vi "Zaber Beginner - Send a List of Commands.vi"() -> ()   [LabVIEW 2020]
doc: "The simplest VI you can write is just a list of commands with no logic. The block diagram makes a request, waits for the response, and then makes the next request until it gets to the end of the list.\nConnect your Zaber device to power and a serial port, then select the serial port on the front panel. Click the Run arrow, and the device will\ntake 5 steps backwards, and then extend back to where it started. The device has to start at least 50000 microsteps away from the home\nposition, so if you receive error response 21, just extend the device before running the VI. All commands are sent to Zaber device number 1."
uses:
  Public/Utility/Request.ctl
  ZaberTSeries.lvlib
panel:
  in  "VISA resource name":refnum<visa-resource-name>
  # "Connect your Zaber device to power and a serial port, then select the\nserial port below. Click the Run arrow above, and the device will\ntake 5 steps backwards, and then extend back to where it started. \nThe device has to start at least 500 microsteps away from the home\nposition, so if you receive error response 21, just extend the device\nbefore running the VI. All commands are sent to Zaber device number 1.\nType Ctrl-E to see how the block diagram is wired."
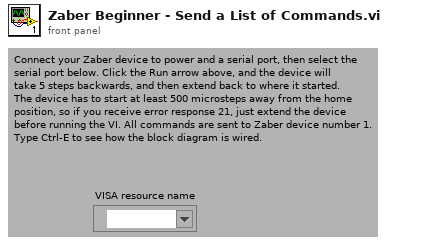
[diagram p1: front panel]
types:
  T1 = typedef "ZaberTSeries.lvlib/Request.ctl" = cluster{"Device Number":u8, "Command":u8, "Data":i32, "Response Count":i32}
  T2 = cluster{"Device Number":u8, "Command":u8, "Data":i32, "Response Count":i32}
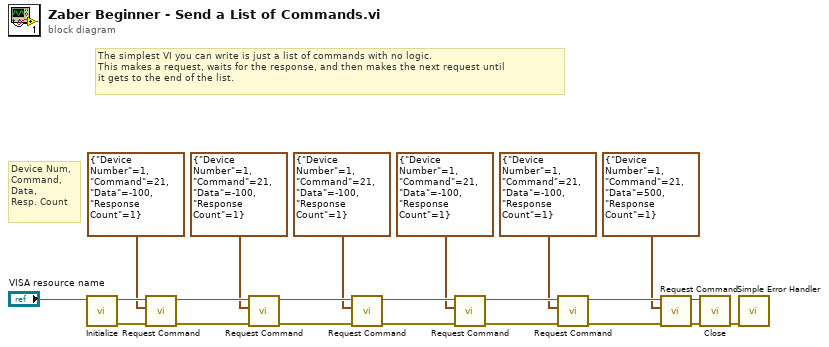
[diagram p0: block diagram]
diagram:
  # "The simplest VI you can write is just a list of commands with no logic.\nThis makes a request, waits for the response, and then makes the next request until\nit gets to the end of the list."
  # "Device Num,\nCommand,\nData,\nResp. Count"
  n1 = call "Initialize.vi"("VISA resource name"="VISA resource name") -> ("error out"=w22:errorcluster, "VISA resource name out"=w19:refnum<visa-resource-name>)  [unwired: 8 in, 1 out]
  n2 = call "Request Command.vi"("error in (no error)"=w22, "Request"=T2 {"Device Number"=1, "Command"=21, "Data"=-100, "Response Count"=1}, "VISA resource name"=w19) -> ("error out"=w21:errorcluster, "VISA resource name out"=w18:refnum<visa-resource-name>)  [unwired: 5 in, 2 out]
  n3 = call "Request Command.vi"("error in (no error)"=w21, "Request"=T1 {"Device Number"=1, "Command"=21, "Data"=-100, "Response Count"=1}, "VISA resource name"=w18) -> ("error out"=w7:errorcluster, "VISA resource name out"=w16:refnum<visa-resource-name>)  [unwired: 5 in, 2 out]
  n4 = call "Request Command.vi"("error in (no error)"=w7, "Request"=T1 {"Device Number"=1, "Command"=21, "Data"=-100, "Response Count"=1}, "VISA resource name"=w16) -> ("error out"=w8:errorcluster, "VISA resource name out"=w15:refnum<visa-resource-name>)  [unwired: 5 in, 2 out]
  n5 = call "Request Command.vi"("error in (no error)"=w8, "Request"=T1 {"Device Number"=1, "Command"=21, "Data"=-100, "Response Count"=1}, "VISA resource name"=w15) -> ("error out"=w9:errorcluster, "VISA resource name out"=w14:refnum<visa-resource-name>)  [unwired: 5 in, 2 out]
  n6 = call "Request Command.vi"("error in (no error)"=w9, "Request"=T1 {"Device Number"=1, "Command"=21, "Data"=-100, "Response Count"=1}, "VISA resource name"=w14) -> ("error out"=w10:errorcluster, "VISA resource name out"=w13:refnum<visa-resource-name>)  [unwired: 5 in, 2 out]
  n7 = call "Request Command.vi"("error in (no error)"=w10, "Request"=T1 {"Device Number"=1, "Command"=21, "Data"=500, "Response Count"=1}, "VISA resource name"=w13) -> ("error out"=w11:errorcluster, "VISA resource name out"=w12:refnum<visa-resource-name>)  [unwired: 5 in, 2 out]
  n8 = call "Close.vi"("error in (no error)"=w11, "VISA resource name"=w12) -> ("error out"=w20:errorcluster)  [unwired: 8 in, 1 out]
  n9 = call <vilib>:"Simple Error Handler.vi"("error in (no error)"=w20) -> ()  [unwired: 4 in, 5 out]
